vi "Model_Destroy.vi"(8 "error in (no error)":errorcluster caption="错误输入（无错误）", 11 "User Management Model 输入":refnum<class "User Management Model.lvclass">) -> (0 "error out":errorcluster caption="错误输出", 2 "error？":bool, 3 "User Management Model 输出":refnum<class "User Management Model.lvclass">)   [LabVIEW 2019, in "User Management Model.lvclass"]
uses:
  User Management Model.lvclass
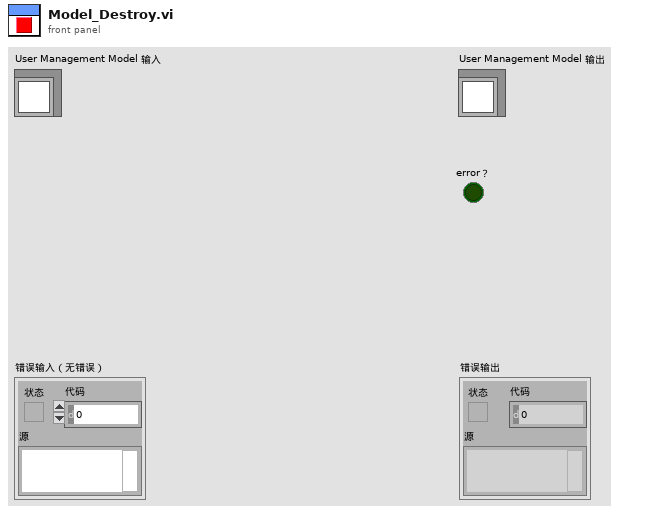
[diagram p1: front panel]
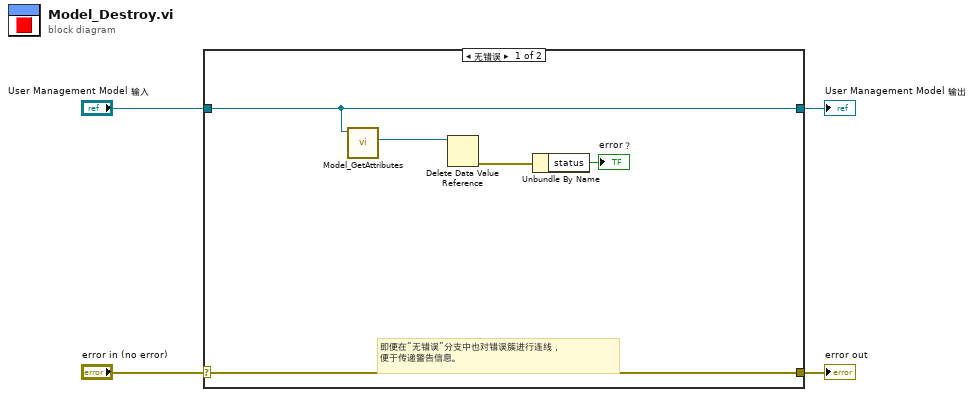
[diagram p0: block diagram]
diagram:
  n1 = case shown="无错误" "error in (no error)" {
    selector: "error in (no error)" -> [w9 w11]
    tunnel: [w9 w11] -> w3
    tunnel: [w8 w10] -> w1
    tunnel: "User Management Model 输入" -> [w8 w10]
    frame No Error {
      # "即便在“无错误”分支中也对错误簇进行连线，\n便于传递警告信息。"
      n2 = call "Model_GetAttributes.vi"("User Management Model 输入"=w8) -> ("属性引用"=w7:refnum<data-value>)  [unwired: 7 in, 3 out]
      n3 = Delete Data Value Reference(data value reference=w7) -> (error out=w6:errorcluster)  [unwired: 1 in, 1 out]
      n4 = Unbundle By Name(w6) -> ("status"=→"error？":bool)
    }
    frame Error {
    }
  }
  "error out" <- w3
  "User Management Model 输出" <- w1
